vi "Configure Control AI Burnout.vi"(0 "VISA resource name":refnum<visa-resource-name>, 5 "Unit No. (0)":i32 min=0 max=6, 7 "Module No.(0)":i32 min=0 max=9, 9 "AI No.(1)":i32=1 min=1 max=2, 11 "error in (no error)":errorcluster, 12 "Burnout Action(0:Off)":i32 min=0 max=2) -> (4 "VISA resource name out":refnum<visa-resource-name>, 6 "AI No.":i32, 8 "Unit No.":i32, 10 "Module No.":i32, 15 "error out":errorcluster)   [LabVIEW 2020, in "Yokogawa GX Series.lvlib"]
doc: "Sets the action of burnout for AI channel in PID mdule.\n\nCommand: SCtrlBurnOut"
uses:
  <instrlib>/Yokogawa GX Series/Yokogawa GX Series.lvlib
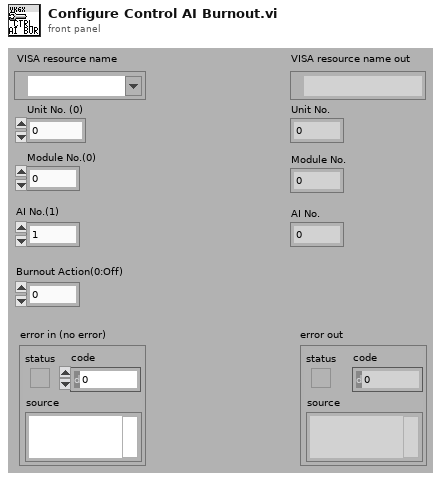
[diagram p1: front panel]
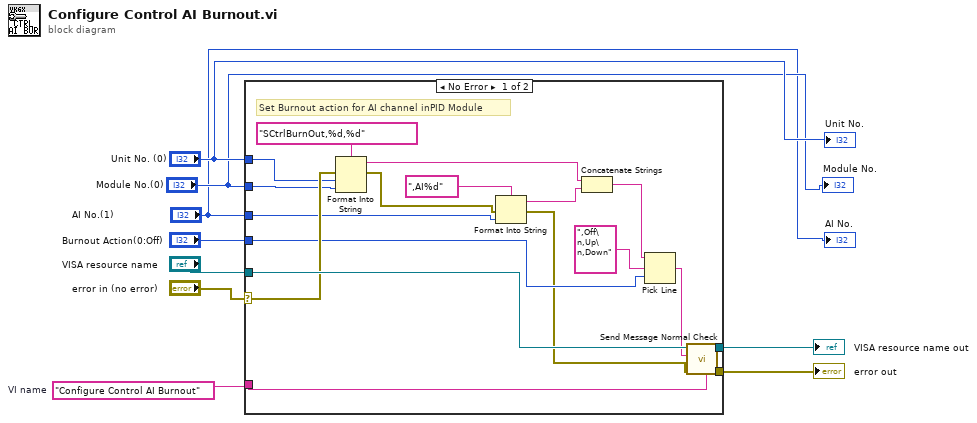
[diagram p0: block diagram]
diagram:
  w5 = "Configure Control AI Burnout"  # VI name
  n1 = case shown="No Error" "error in (no error)" {
    selector: "error in (no error)" -> [w23 w28]
    tunnel: [w27 w29] -> w9
    tunnel: [w26 w28] -> w8
    tunnel: "VISA resource name" -> [w25 w29]
    tunnel: w5 -> [w22 _]
    tunnel: "Unit No. (0)" -> [w18 _]
    tunnel: "Module No.(0)" -> [w17 _]
    tunnel: "Burnout Action(0:Off)" -> [w20 _]
    tunnel: "AI No.(1)" -> [w15 _]
    frame No Error {
      # "Set Burnout action for AI channel inPID Module"
      n2 = Format Into String(format string="SCtrlBurnOut,%d,%d", error in=w23, w18, w17) -> (resulting string=w12:string, error out=w14:errorcluster)  [unwired: 1 in]
      n3 = Format Into String(format string=",AI%d", error in=w14, w15) -> (resulting string=w11:string, error out=w13:errorcluster)  [unwired: 1 in]
      n4 = Concatenate Strings(w12, w11) -> (w10:string)
      n5 = Pick Line(string ("")=w10, multi-line string=",Off\n,Up\n,Down", line index=w20) -> (output string=w19:string)
      n6 = call <instrlib>:"Send Message Normal Check.vi"("Source (\"\")"=w22, "error in (no error)"=w13, "Send Message (\"\")"=w19, "VISA resource name"=w25) -> ("error out"=w26:errorcluster, "VISA resource name out"=w27:refnum<visa-resource-name>)  [unwired: 2 in, 4 out]
    }
    frame Error {
    }
  }
  "error out" <- w8
  "VISA resource name out" <- w9
  "Unit No." <- "Unit No. (0)"
  "Module No." <- "Module No.(0)"
  "AI No." <- "AI No.(1)"
